vi "PXI_Health_WhiteScreen_Test.vi"() -> ()   [LabVIEW 2018]
panel:
  out "Numeric":i32
  out "error out":errorcluster
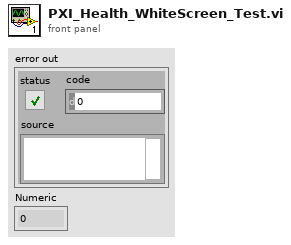
[diagram p1: front panel]
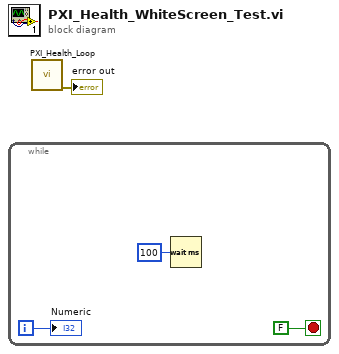
[diagram p0: block diagram]
diagram:
  n1 = while {
    i -> [w3]
    stop <- FALSE stop-if-true
    n2 = Wait (ms)(milliseconds to wait=u32 100) -> ()  [unwired: 1 out]
    "Numeric" <- w3
  }
  n3 = call "PXI_Health_Loop.vi"() -> ("error out"=→"error out":errorcluster)  [unwired: 11 in]
